vi "TextDocument_GetStyleByName.vi"(8 "error in":errorcluster, 10 "StyleName":string, 11 "TextDocument in":refnum<k24>) -> (0 "error out":errorcluster, 2 "Style":refnum<k24>, 3 "TextDocument out":refnum<k24>)   [LabVIEW 2009]
uses:
  C:/Projets/LAVAG/OpenOfficeRGT/AODL/DLLs/AODL.dll
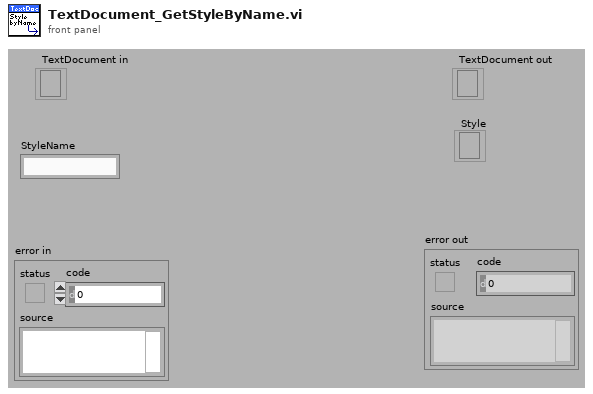
[diagram p1: front panel]
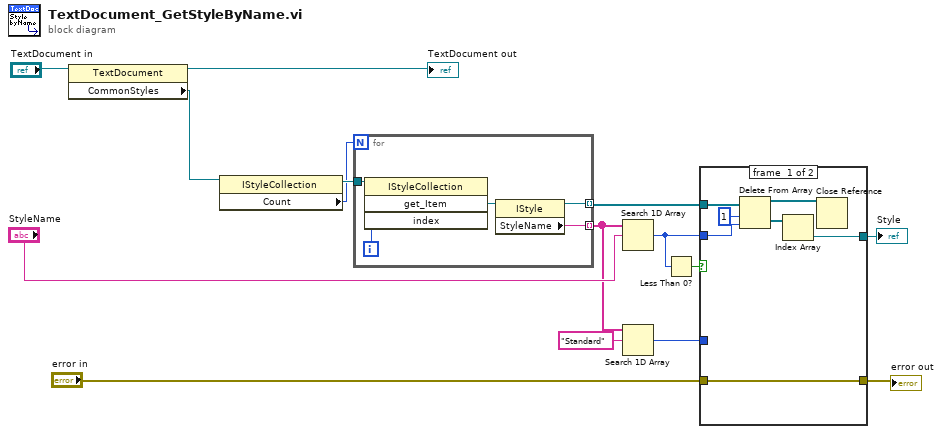
[diagram p0: block diagram]
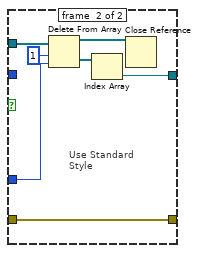
[diagram p2: hidden frame]
diagram:
  n1 = property class="TextDocument"(reference="TextDocument in") -> (reference out=→"TextDocument out":refnum<k24>, "CommonStyles"=w13:refnum<k24>)  [unwired: 1 in, 1 out]
  n2 = property class="IStyleCollection"(reference=w13) -> (reference out=w12:refnum<k24>, "Count"=w11:i32)  [unwired: 1 in, 1 out]
  n3 = for {
    N: w11 -> [_]
    tunnel: w12 -> [w20]
    tunnel: [w17] -> w3 mode=indexing
    tunnel: [w16] -> w9 mode=indexing
    i -> [w19]
    n4 = invoke class="IStyleCollection" method="get_Item"(reference=w20, "index"=w19) -> ("get_Item"=w18:refnum<k24>)  [unwired: 2 in, 3 out]
    n5 = property class="IStyle"(reference=w18) -> (reference out=w16:refnum<k24>, "StyleName"=w17:string)  [unwired: 1 in, 1 out]
  }
  n6 = Search 1D Array(1D array=w3, element="StyleName") -> (index of element=w7:i32)  [unwired: 1 in]
  n7 = Search 1D Array(1D array=w3, element="Standard") -> (index of element=w1:i32)  [unwired: 1 in]
  n8 = Less Than 0?(x=w7) -> (x < 0?=w6:bool)
  n9 = case shown="True" w6 {
    tunnel: w9 -> [w27 w34]
    tunnel: [w24 w31] -> w8
    tunnel: w7 -> [w22 _]
    tunnel: "error in" -> [w21 w29]
    tunnel: [w21 w29] -> w4
    tunnel: w1 -> [_ w28]
    frame #0 {
      n10 = Delete From Array(array=w27, length=1, index=w22) -> (deleted portion=w25:refnum<k24>[], array with subset deleted=w23:refnum<k24>[])
      n11 = Index Array(array=w25) -> (element=w24:refnum<k24>)  [unwired: 1 in]
      n12 = Close Reference(reference=w23) -> ()  [unwired: 1 in, 1 out]
    }
    frame #1 {
      # "Use Standard\nStyle"
      n13 = Delete From Array(array=w34, length=1, index=w28) -> (deleted portion=w32:refnum<k24>[], array with subset deleted=w30:refnum<k24>[])
      n14 = Index Array(array=w32) -> (element=w31:refnum<k24>)  [unwired: 1 in]
      n15 = Close Reference(reference=w30) -> ()  [unwired: 1 in, 1 out]
    }
  }
  "error out" <- w4
  "Style" <- w8
